vi "Load From Panel Layout File.vi"(8 "error in":errorcluster, 11 "panel layout file":path) -> (0 "error out":errorcluster, 3 "panel layout out":refnum<class "VI Panel Layout.lvclass">)   [LabVIEW 2012, in "NI_SE_Front Panel Layout.lvlib" / "VI Panel Layout.lvclass"]
doc: "Load a panel layout description from disk."
uses:
  VI Panel Layout.lvclass
  VI Panel Layout.lvclass/VI Panel Layout.ctl
  Object Layout Classes/Object Layout/Object Layout.lvclass/Object Layout.ctl
  Object Layout Classes/Object Layout/Get UID.vi
  Object Layout Classes/Object Layout/Get Unique Name.vi
  Convert UID To String.vi
  NI_SE_Front Panel Layout.lvlib
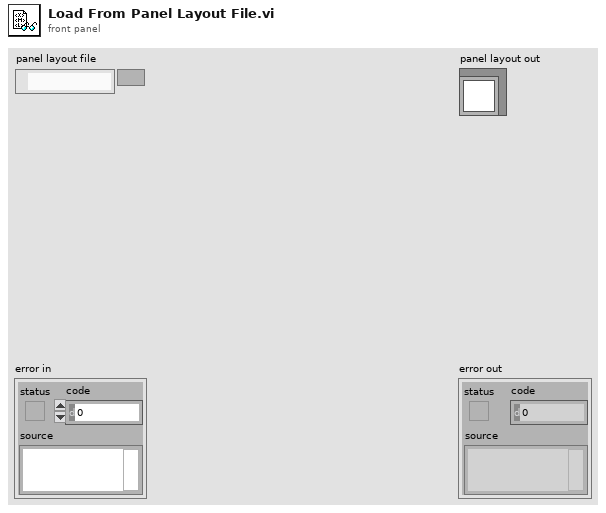
[diagram p1: front panel]
types:
  T1 = enum16{"open", "replace", "create", "open or create", "replace or create", "replace or create with confirmation"}
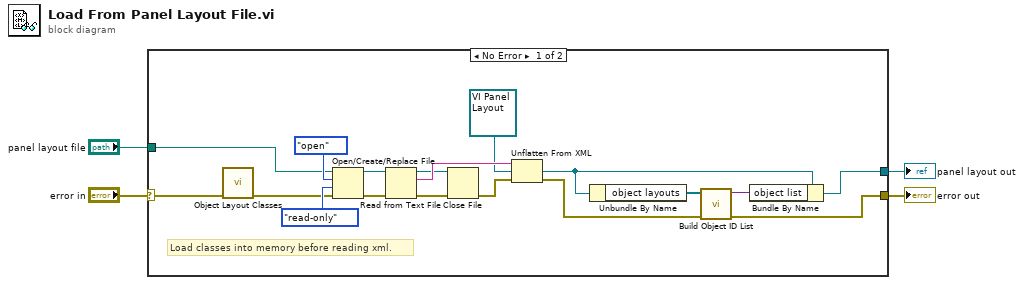
[diagram p0: block diagram]
diagram:
  n1 = case shown="No Error" "error in" {
    selector: "error in" -> [w22 w23]
    tunnel: [w7 w23] -> w3
    tunnel: [w9 _] -> w2
    tunnel: "panel layout file" -> [w12 _]
    frame No Error {
      # "Load classes into memory before reading xml."
      n2 = call "Object Layout Classes.vi"("error in"=w22) -> ("error out"=w13:errorcluster)  [unwired: 9 in, 1 out]
      n3 = Open/Create/Replace File(file path (use dialog)=w12, error in=w13, operation (0:open)=T1."open", access (0:read/write)=enum16{"read/write", "read-only", "write-only"}."read-only") -> (refnum out=w5:refnum<file>, error out=w17:errorcluster)  [unwired: 2 in, 1 out]
      n4 = Read from Text File(file (use dialog)=w5, error in=w17) -> (refnum out=w18:refnum<file>, text=w20:string, error out=w19:errorcluster)  [unwired: 2 in, 1 out]
      n5 = Close File(refnum=w18, error in=w19) -> (error out=w21:errorcluster)  [unwired: 1 out]
      n6 = Unflatten From XML(xml string=w20, type=refnum<class "VI Panel Layout.lvclass"> refnum ("VI Panel Layout out"), error in (no error)=w21) -> (value=w6:refnum<class "VI Panel Layout.lvclass">, error out=w8:errorcluster)
      n7 = Unbundle By Name(w6) -> ("object layouts"=w11:refnum<class "Object Layout.lvclass">[])
      n8 = call "Build Object ID List.vi"("error in"=w8, "object layouts"=w11) -> ("error out"=w7:errorcluster, "object ID list"=w10:variant)  [unwired: 8 in]
      n9 = Bundle By Name(cluster=w6, "object list"=w10) -> (w9:refnum<class "VI Panel Layout.lvclass">)
    }
    frame Error {
    }
  }
  "error out" <- w3
  "panel layout out" <- w2
